vi "Nulldetector.vi"(7 "Readings (10)":i32=10, 8 "error in (no error)":errorcluster) -> (0 "error out":errorcluster, 2 "Voltages (V)":dbl[](array[numeric]) format="%#_9g", 3 "Relative times (s)":dbl[](array[numeric]) format="%#_9g")   [LabVIEW 2019, in "ACSVcontrol-driver.lvlib"]
doc: "Returns readings from the nulldetector. This VI is not finished and is missing some possibilities."
uses:
  ACSVcontrol-driver.lvlib
  Private/Type definitions/Command.ctl
  Private/Type definitions/Status.ctl
  Private/Type definitions/Instruction.ctl
  Private/Globals.vi
  <vilib>/Utility/error.llb/Error Cluster From Error Code.vi
  <vilib>/ErrorRing/Error Ring.xnode
panel:
  out "Mean (V)":dbl
  out "Std. Dev. (V)":dbl
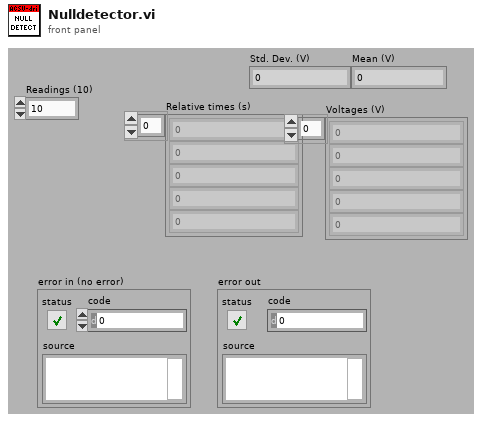
[diagram p1: front panel]
types:
  T1 = typedef "ACSVcontrol-driver.lvlib/Status.ctl" = enum16{"waiting", "processing", "error command", "Set_PJVS-Done", "Set_Mux-Done", "Set_Mux-Error", "Set_57XX-Done", "Set_57XX-Error", "Set_Gen-Done", "Set_Gen-Error", "Set_Synthesizer-Done", "Set_Synthesizer-Error", "Read_Nano-Done", "Read_Sampler-Done", "Read_Sampler-Error", "Read_Sensors-Done"}
  T2 = typedef "ACSVcontrol-driver.lvlib/Command.ctl" = enum16{"Set_PJVS", "Set_Mux", "Set_57XX", "Set_Gen", "Set_Synthesizer", "Read_Nulldetector", "Read_Sampler", "Read_Sensors"}
  T3 = typedef "ACSVcontrol-driver.lvlib/Instruction.ctl" = enum16{"dummy - do not use", "Send Command", "Read Result", "Ask Status"}
  T4 = typedef "ACSVcontrol-driver.lvlib/Timeouts.ctl" = cluster{"TCP Read & Write (ms)":i32, "Sensors readout":i32, "PJVS setup":i32, "Nullmeter readout":i32, "Multiplexer setup":i32, "57XX setup":i32, "Generator setup":i32, "Synthesizer setup":i32, "Sampler readout":i32}
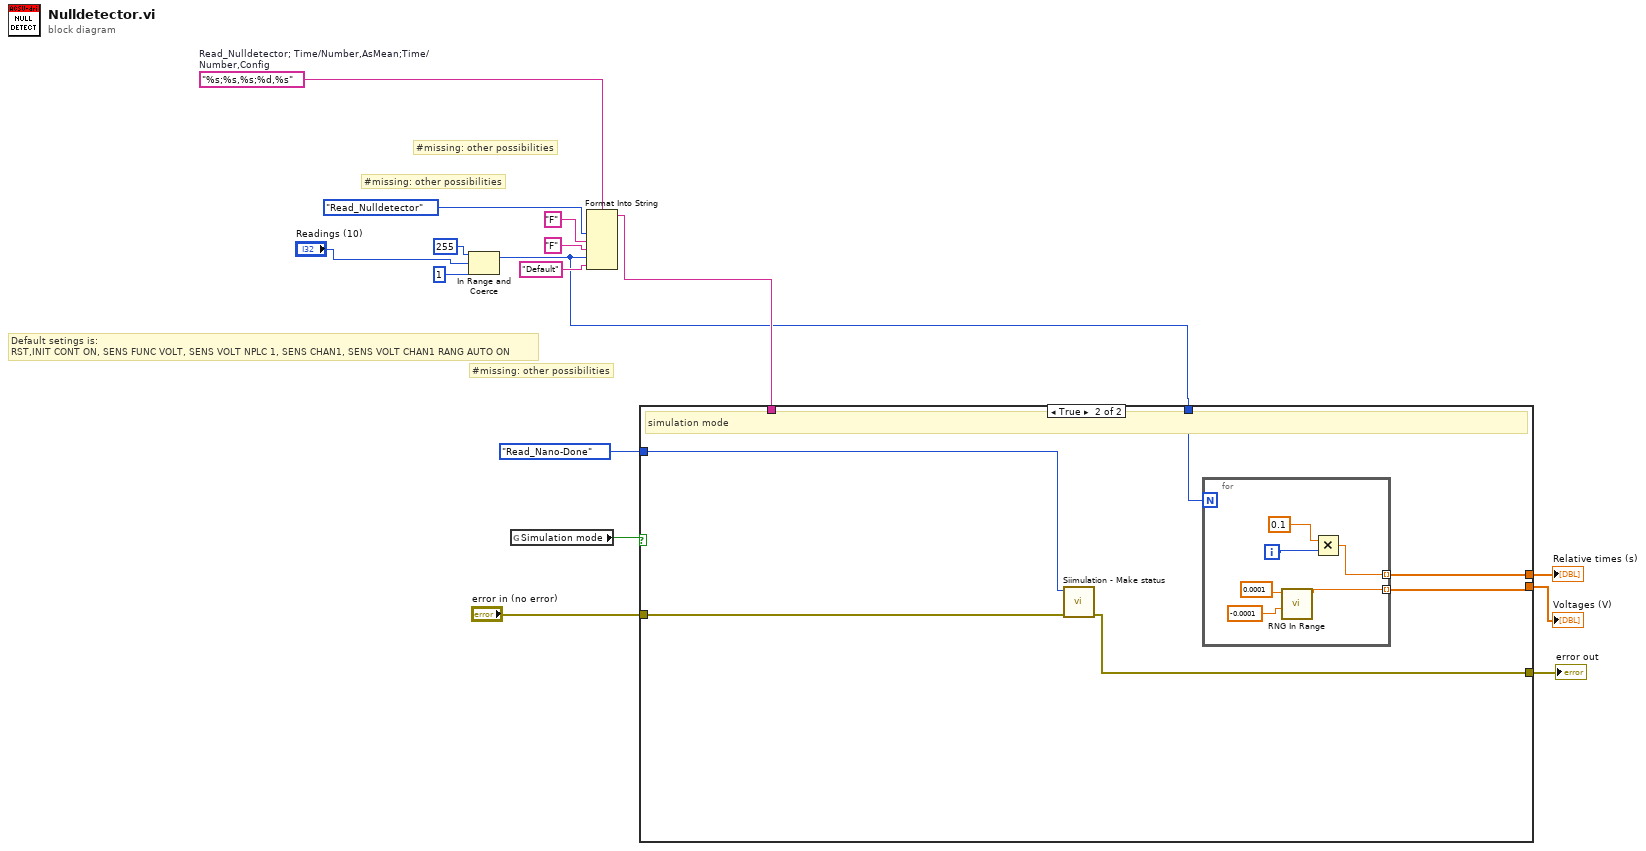
[diagram p0: block diagram]
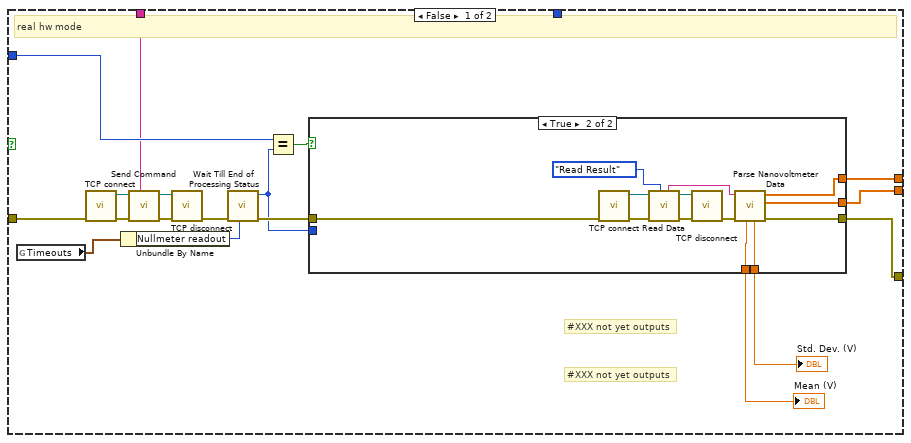
[diagram p2: hidden frame]
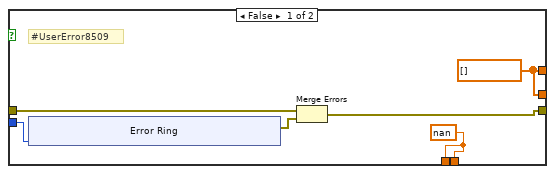
[diagram p3: hidden frame]
diagram:
  w16 = "%s;%s,%s;%d,%s"  # Read_Nulldetector; Time/Number,AsMean;Time/Number,Config
  # "Default setings is:\nRST,INIT CONT ON, SENS FUNC VOLT, SENS VOLT NPLC 1, SENS CHAN1, SENS VOLT CHAN1 RANG AUTO ON"
  # "#missing: other possibilities"
  # "#missing: other possibilities"
  # "#missing: other possibilities"
  n1 = In Range and Coerce(upper limit=255, x="Readings (10)", lower limit=1) -> (coerced(x)=w2:i32)  [unwired: 1 out]
  n2 = global read "Globals.vi" "Simulation mode"() -> (w1:bool)
  n3 = Format Into String(format string=w16, Command."Read_Nulldetector" ("Command"), "F" ("resulting string"), "F" ("resulting string"), w2, "Default" ("input 5")) -> (resulting string=w3:string)  [unwired: 2 in, 1 out]
  n4 = case shown="True" w1 {
    tunnel: "error in (no error)" -> [w34 w66]
    tunnel: Status."Read_Nano-Done" ("x") -> [w28 w64]
    tunnel: [w24 w65] -> w6
    tunnel: [w23 w62] -> w5
    tunnel: [w22 w61] -> w4
    tunnel: w3 -> [w19 _]
    tunnel: w2 -> [_ w63]
    frame False {
      # "#XXX not yet outputs"
      # "#XXX not yet outputs"
      # "real hw mode"
      n5 = global read "Globals.vi" "Timeouts"() -> (w20:T4)
      n6 = call "TCP connect.vi"("error in (no error)"=w34) -> ("error out"=w33:errorcluster, "connection ID"=w32:refnum<k5>)  [unwired: 9 in]
      n7 = Unbundle By Name(w20) -> ("Nullmeter readout"=w21:i32)
      n8 = call "Send Command.vi"("Command"=w19, "error in (no error)"=w33, "connection ID"=w32) -> ("error out"=w31:errorcluster, "connection ID out"=w30:refnum<k5>)  [unwired: 7 in]
      n9 = call "TCP disconnect.vi"("error in (no error)"=w31, "connection ID"=w30) -> ("error out"=w25:errorcluster)  [unwired: 9 in]
      n10 = call "Wait Till End of Processing Status.vi"("Loop Timeout (ms) (5000)"=w21, "error in (no error)"=w25) -> ("error out"=w29:errorcluster, "Last Status"=w26:T1)  [unwired: 8 in]
      n11 = Equal?(x=w28, y=w26) -> (x = y?=w27:bool)
      n12 = case shown="True" w27 {
        tunnel: w29 -> [w40 w58]
        tunnel: [w37 w54] -> w24
        tunnel: w26 -> [w39 _]
        tunnel: [w36 w53] -> w23
        tunnel: [w36 w52] -> w22
        tunnel: [w35 w49] -> w18
        tunnel: [w35 w48] -> w17
        frame False {
          w35 = nan
          w36 = dbl[] [] ("Relative times (s)")
          # "#UserError8509"
          n13 = xnode "Error Ring"("parameter 0"=w39) -> ("error out"=w38:errorcluster)
          n14 = Merge Errors(w40, w38) -> (w37:errorcluster)
        }
        frame True {
          n15 = call "TCP connect.vi"("error in (no error)"=w58) -> ("error out"=w57:errorcluster, "connection ID"=w56:refnum<k5>)  [unwired: 9 in]
          n16 = call "Read Data.vi"("Instruction"=Instruction."Read Result", "error in (no error)"=w57, "connection ID"=w56) -> ("error out"=w60:errorcluster, "connection ID out"=w59:refnum<k5>, "Data"=w50:string)  [unwired: 6 in]
          n17 = call "TCP disconnect.vi"("error in (no error)"=w60, "connection ID"=w59) -> ("error out"=w55:errorcluster)  [unwired: 9 in]
          n18 = call "Parse Nanovoltmeter Data.vi"("error in"=w55, "Data"=w50) -> ("error out"=w54:errorcluster, "Voltages (V)"=w52:dbl[], "Relative times (s)"=w53:dbl[], "Std. Dev. (V)"=w49:dbl, "Mean (V)"=w48:dbl)  [unwired: 5 in]
        }
      }
      "Std. Dev. (V)" <- w18
      "Mean (V)" <- w17
    }
    frame True {
      # "simulation mode"
      n19 = call "Siimulation - Make status.vi"("error in (no error)"=w66, "Status"=w64) -> ("error out"=w65:errorcluster)  [unwired: 8 in, 1 out]
      n20 = for {
        N: w63 -> [_]
        tunnel: [w70] -> w62 mode=indexing
        tunnel: [w69] -> w61 mode=indexing
        i -> [w72]
        n21 = call "RNG In Range.vi"("llimit 2 (1)"=-0.0001 ("upper bound (100)"), "limit 1 (0)"=0.0001 ("upper bound (100)")) -> ("number"=w69:dbl)  [unwired: 9 in]
        n22 = Multiply(x=0.1, y=w72) -> (x*y=w70:dbl)
      }
    }
  }
  "error out" <- w6
  "Relative times (s)" <- w5
  "Voltages (V)" <- w4
